vi "Num2Fieldstring.vi"(10 "String":string="Z: ", 11 "In":dbl format="%#_13g") -> (3 "Out":string)   [LabVIEW 2018]
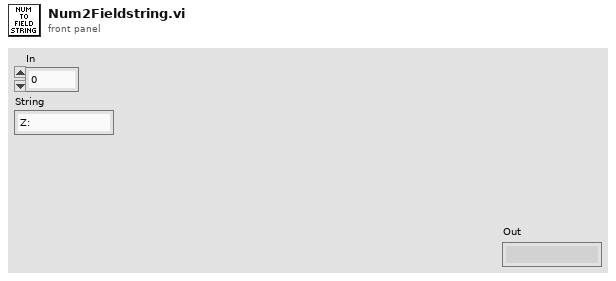
[diagram p1: front panel]
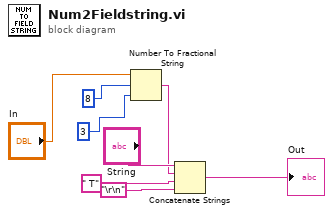
[diagram p0: block diagram]
diagram:
  n1 = Number To Fractional String(number="In", width (-)=8, precision (6)=3) -> (F-format string=w4:string)  [unwired: 1 in]
  n2 = Concatenate Strings("String", w4, " T", "\r\n") -> (→"Out":string)
